vi "RegReadExtLong UnitTest.vi"() -> ()   [LabVIEW 2018]
uses:
  Downloads/MIPI RFFE API/Controls/RFFE Commands Type Def.ctl
  Downloads/MIPI RFFE API/Controls/Write Data Strict Type Def.ctl
  Command/RFFE Command.lvclass
  RegReadExtLong/RFFE RegReadExtLong Command.lvclass
  C:/Users/semoore/Projects/mipi-rffe-labview-oop/Command/RFFE Command.lvclass
panel:
  out "arrays same size?":bool
  out "data equal?":bool
  out "error in (no error) 2":errorcluster
  in  "error in (no error)":errorcluster
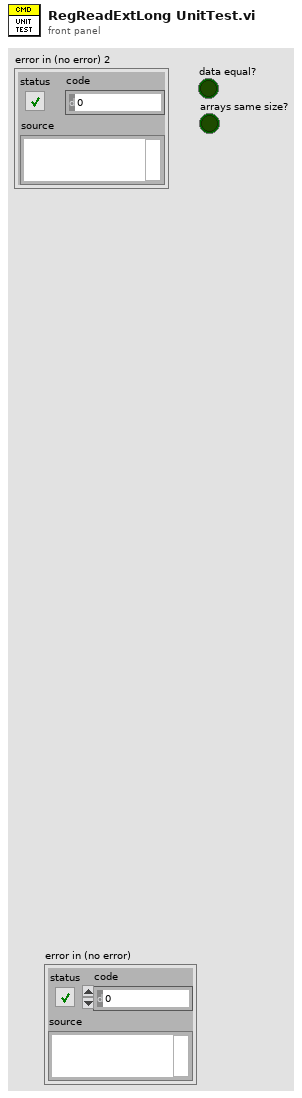
[diagram p1: front panel]
types:
  T1 = typedef "Write Data Strict Type Def.ctl" = cluster{"slave address":u8, "register address":u16, "register data (write)":u8[], "byte count":u8}
  T2 = typedef "RFFE Commands Type Def.ctl" = enum16{"Reg0Write", "RegWrite", "RegRead", "RegReadHR", "RegWriteExt", "RegReadExt", "RegReadExtHR", "RegWriteExtLong", "RegReadExtLong", "RegReadExtLongHR"}
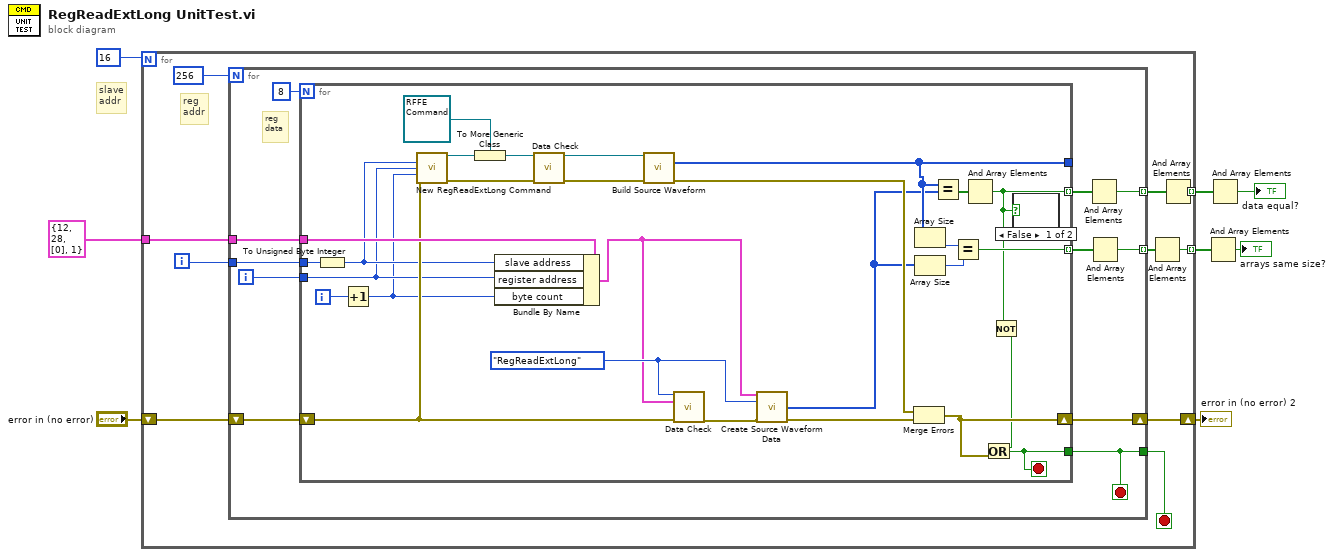
[diagram p0: block diagram]
diagram:
  # "slave\naddr"
  n1 = for {
    N: 16 -> [_]
    tunnel: T1 {"slave address"=12, "register address"=28, "register data (write)"=[0], "byte count"=1} ("Register Data") -> [w17]
    shift-right: [w14] -> w5
    shift-left: "error in (no error)" -> [w18]
    tunnel: [w12] -> w4 mode=indexing
    tunnel: [w10] -> w2 mode=indexing
    i -> [w16]
    stop <- w9 stop-if-true
    # "reg\naddr"
    n2 = for {
      N: 256 -> [_]
      tunnel: w17 -> [w28]
      tunnel: w16 -> [w25]
      shift-right: [w24] -> w14
      shift-left: w18 -> [w29]
      tunnel: [w22] -> w13 mode=indexing
      tunnel: [w20] -> w11 mode=indexing
      tunnel: [w19] -> w9
      i -> [w26]
      stop <- w19 stop-if-true
      # "reg\ndata"
      n3 = for {
        N: 8 -> [_]
        tunnel: w28 -> [w55]
        tunnel: [w38] -> _
        tunnel: w26 -> [w32]
        tunnel: w25 -> [w44]
        shift-right: [w48] -> w24
        shift-left: w29 -> [w45]
        tunnel: [w36] -> w23 mode=indexing
        tunnel: [w39] -> w21 mode=indexing
        tunnel: [w35] -> w19
        i -> [w31]
        stop <- w35 stop-if-true
        w57 = RFFE_Commands_Type_Def."RegReadExtLong" ("RFFE command")
        n4 = To Unsigned Byte Integer(number=w44) -> (unsigned 8bit integer=w33:u8)
        n5 = Increment(x=w31) -> (x+1=w30:i32)
        n6 = call "New RegReadExtLong Command.vi"("Slave Address"=w33, "Register Address"=w32, "Byte Count"=w30, "error in (no error)"=w45) -> ("RFFE RegReadExtLong Command out"=w51:refnum<class "RFFE RegReadExtLong Command.lvclass">, "error out"=w52:errorcluster)  [unwired: 10 in]
        n7 = To More Generic Class(target class=refnum<class "RFFE Command.lvclass"> refnum ("RFFE Commands.lvlib:RFFE Command.lvclass"), reference=w51) -> (generic class reference=w41:refnum<class "RFFE Command.lvclass">)
        n8 = Bundle By Name(cluster=w55, "slave address"=w33, "register address"=w32, "byte count"=w30) -> (w54:T1)
        n9 = call-dynamic "Data Check.vi"("RFFE Command in"=w41, "error in (no error)"=w52) -> ("RFFE Command out"=w50:refnum<class "RFFE Command.lvclass">, "error out"=w53:errorcluster)  [unwired: 12 in]
        n10 = call-dynamic "Build Source Waveform.vi"("RFFE Command in"=w50, "error in (no error)"=w53) -> ("Source Waveform"=w38:u32[], "error out"=w47:errorcluster)  [unwired: 11 in, 1 out]
        n11 = call "Data Check.vi"("RFFE command"=w57, "Register Data"=w54, "error in"=w45) -> ("error out"=w56:errorcluster)  [unwired: 12 in]
        n12 = call "Create Source Waveform Data.vi"("Register Data"=w54, "RFFE command"=w57, "error in"=w56) -> ("RFFEWrite source waveform data array"=w37:u32[], "error out"=w49:errorcluster)  [unwired: 10 in, 1 out]
        n13 = Merge Errors(w47, w49) -> (w48:errorcluster)
        n14 = Array Size(array=w38) -> (size(s)=w43:i32)
        n15 = Array Size(array=w37) -> (size(s)=w42:i32)
        n16 = Equal?(x=w38, y=w37) -> (x = y?=w46:bool[])
        n17 = Equal?(x=w43, y=w42) -> (x = y?=w39:bool)
        n18 = And Array Elements(Boolean array=w46) -> (logical AND=w36:bool)
        n19 = Not(x=w36) -> (.not. x?=w34:bool)
        n20 = Or(x=w34, y=w48) -> (x .or. y?=w35:bool)
        n21 = case shown="False" w36 {
          frame False {
          }
          frame True {
          }
        }
      }
      n22 = And Array Elements(Boolean array=w23) -> (logical AND=w22:bool)
      n23 = And Array Elements(Boolean array=w21) -> (logical AND=w20:bool)
    }
    n24 = And Array Elements(Boolean array=w11) -> (logical AND=w10:bool)
    n25 = And Array Elements(Boolean array=w13) -> (logical AND=w12:bool)
  }
  "error in (no error) 2" <- w5
  n26 = And Array Elements(Boolean array=w2) -> (logical AND=→"arrays same size?":bool)
  n27 = And Array Elements(Boolean array=w4) -> (logical AND=→"data equal?":bool)
